vi "GetFormat.vi"(8 "Error In":errorcluster, 11 "Keithley 6485 In":refnum<visa-resource-name>) -> (0 "Error Out":errorcluster, 2 "Format Elements":T1[](array[typedef]), 3 "Keithley 6485 Out":refnum<visa-resource-name>)   [LabVIEW 2012, in "Keithley-6485.lvlib"]
uses:
  Keithley-6485.lvlib
  Controls/FormatElement.ctl
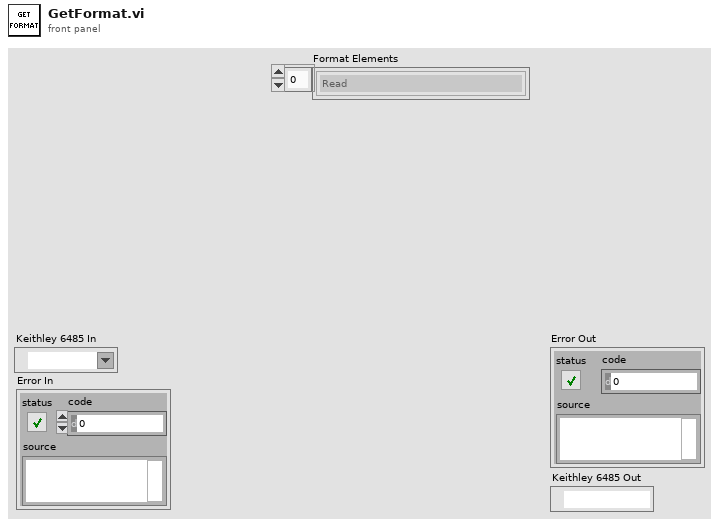
[diagram p1: front panel]
types:
  T1 = typedef "Keithley-6485.lvlib/FormatElement.ctl" = enum16{"Read", "Unit", "Time", "Status"}
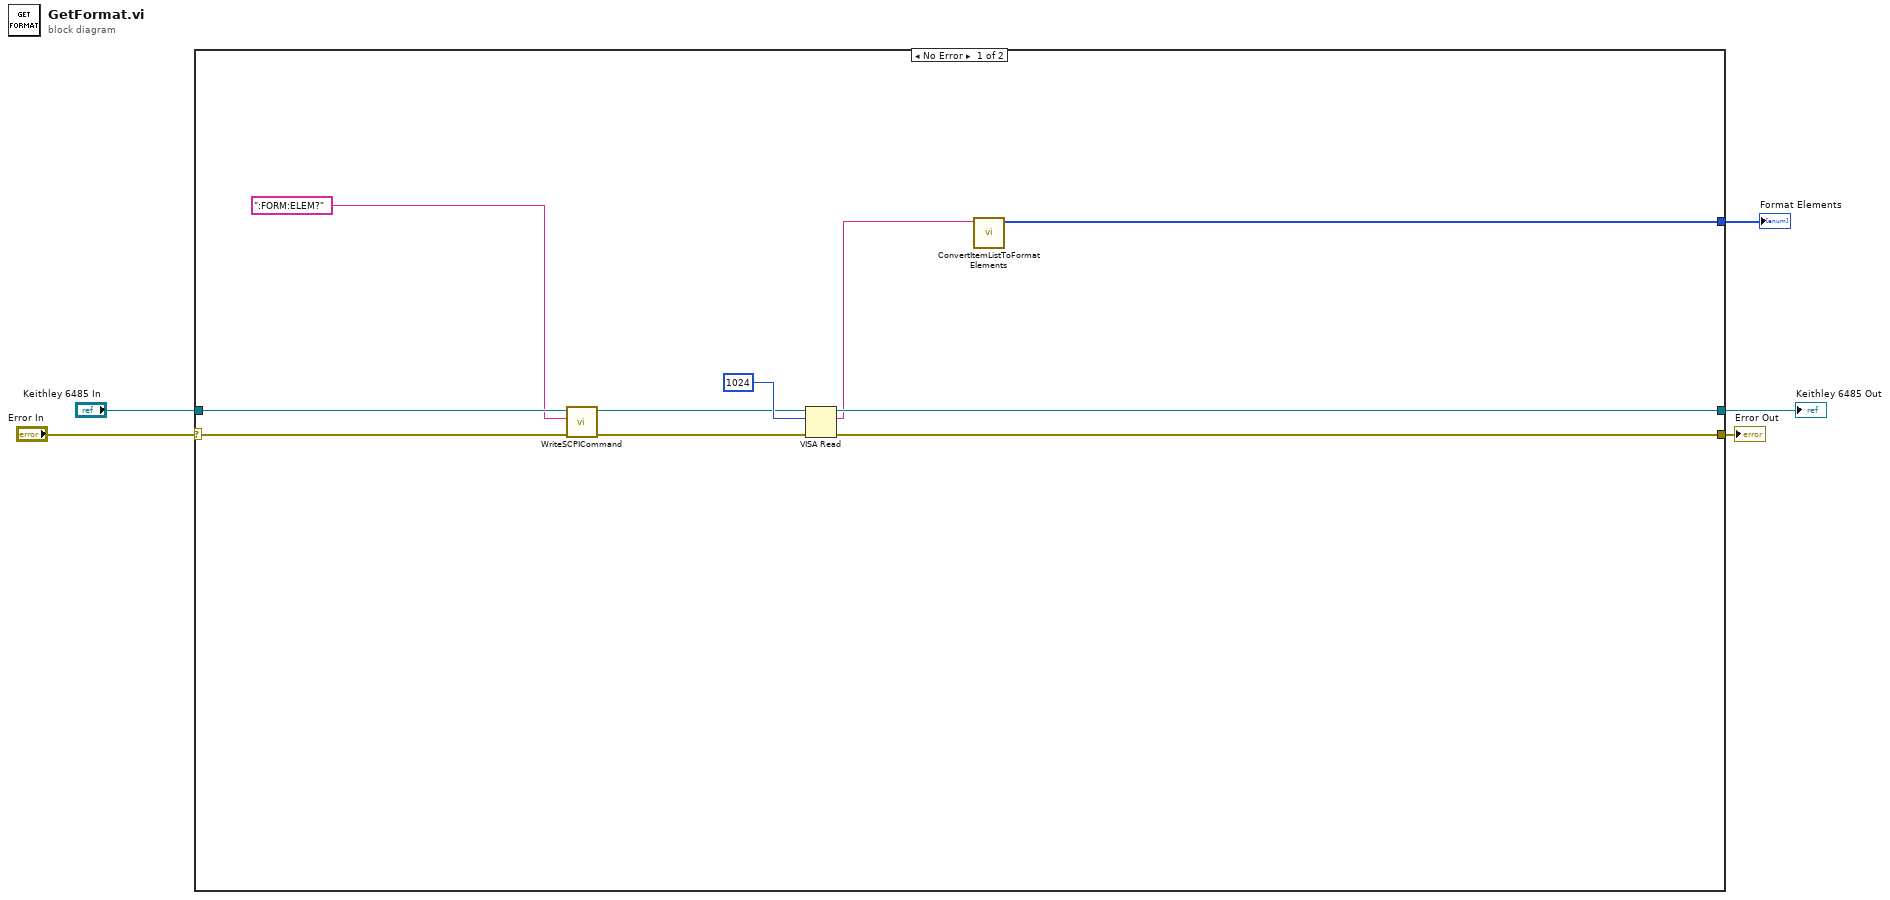
[diagram p0: block diagram]
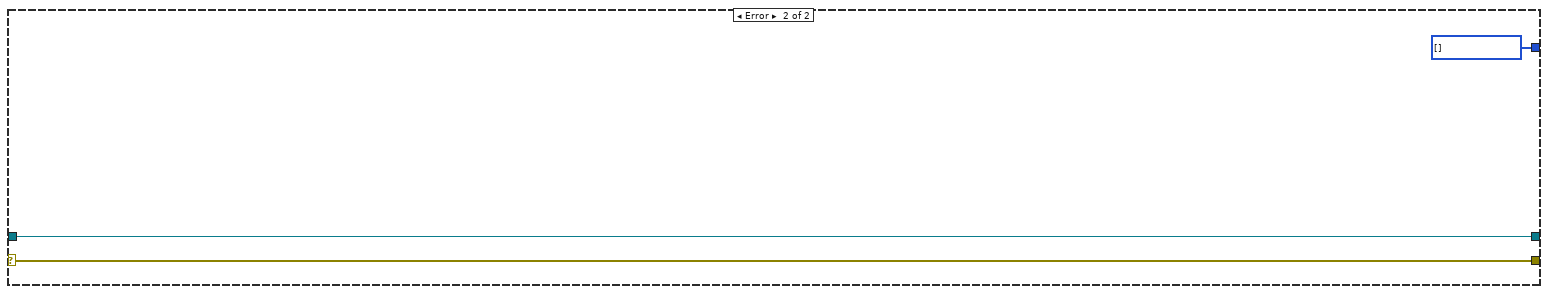
[diagram p2: hidden frame]
diagram:
  n1 = case shown="No Error" "Error In" {
    selector: "Error In" -> [w10 w17]
    tunnel: "Keithley 6485 In" -> [w9 w18]
    tunnel: [w15 w17] -> w3
    tunnel: [w14 w18] -> w2
    tunnel: [w6 w16] -> w1
    frame No Error {
      n2 = call "WriteSCPICommand.vi"("Error In"=w10, "SCPI Command"=":FORM:ELEM?", "Keithley 6482 In"=w9) -> ("Error Out"=w11:errorcluster, "Keithley 6482 Out"=w12:refnum<visa-resource-name>)  [unwired: 7 in]
      n3 = VISA Read(VISA resource name=w12, byte count=u32 1024, error in (no error)=w11) -> (VISA resource name out=w14:refnum<visa-resource-name>, read buffer=w7:string, error out=w15:errorcluster)  [unwired: 1 out]
      n4 = call "ConvertItemListToFormatElements.vi"("Item List"=w7) -> ("Format Elements"=w6:T1[])  [unwired: 10 in]
    }
    frame Error {
      w16 = T1[] [] items=["Read", "Unit", "Time", "Status"] ("Sense Format Elements")
    }
  }
  "Error Out" <- w3
  "Keithley 6485 Out" <- w2
  "Format Elements" <- w1
